vi "PathPlanner_ObstacleGrid_ReadNavFile.vi"(11 "FileName":string="default_navgrid.json") -> (0 "error out":errorcluster, 2 "NavGridObstacles":T1[](array[typedef]), 3 "PathPlanner_Grid":T2, 4 "Full Filename":string)   [LabVIEW 2019, in "PathPlanner24.lvlib"]
doc: "Load an obstacle grid from a JSON formatted file. \n\nInputs: \n - filename - string - The name of the obstacle grid file. See notes below on file naming.\n\nOutputs:\n - PathPlanner_ObstacleGrid - cluster - Obstacle grid read from JSON file.\n - Error out - cluster - Error cluster\n - Full Filename - string - fully qualified file name.\n\nNotes on file naming:\n - The file name must include the extention. \".json\" is not automatically appended to the name. \n - The file name can be a simple file or an absolute path. If a simple file name is used the default path on the RoboRIO is: \"home:\\lvuser\\natinst\\LabVIEW Data\". On a Windows PC the default path is the LabVIEW default directory. Normally this is: “%HOMEDRIVE%%HOMEPATH%\\Documents\\LabView Data\".\n - Filenames on the RoboRIO, which runs Linux, are case sensitive.\ni"
uses:
  PathPlanner24.lvlib
  TypeDef/PathPlannerObstacleGrid.ctl
  TypeDef/PathPlannerFinderGridPosition.ctl
panel:
  in  "error in (no error)":errorcluster
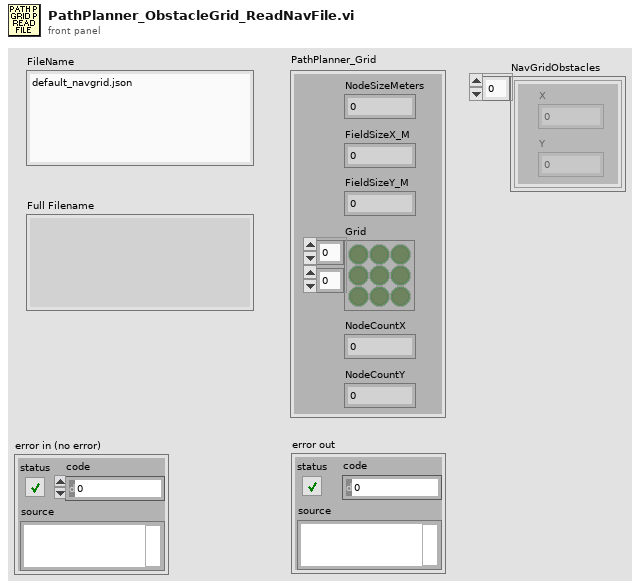
[diagram p1: front panel]
types:
  T1 = typedef "PathPlanner24.lvlib/PathPlannerFinderGridPosition.ctl" = cluster{"X":i32, "Y":i32}
  T2 = typedef "PathPlanner24.lvlib/PathPlannerObstacleGrid.ctl" = cluster{"NodeSizeMeters":dbl, "Grid":bool[][], "NodeCountX":i32, "NodeCountY":i32, "FieldSizeX_M":dbl, "FieldSizeY_M":dbl}
  T3 = enum16{"open", "replace", "create", "open or create", "replace or create", "replace or create with confirmation"}
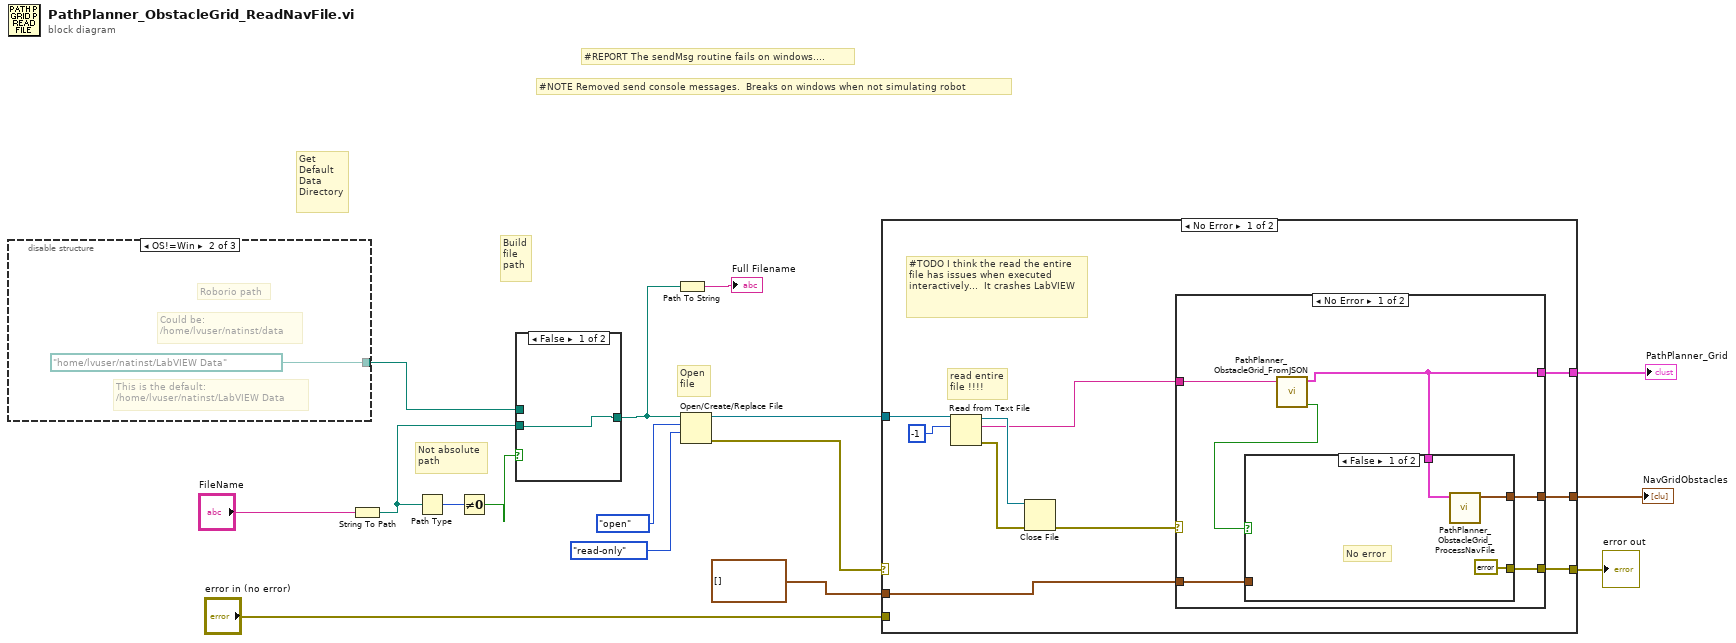
[diagram p0: block diagram]
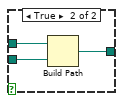
[diagram p2: hidden frame]
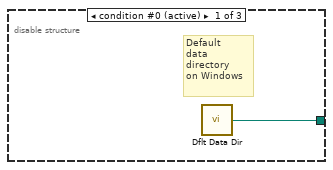
[diagram p3: hidden frame]
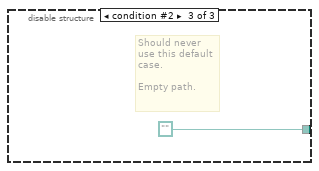
[diagram p4: hidden frame]
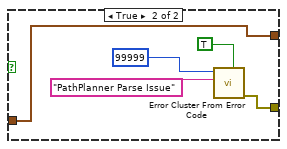
[diagram p5: hidden frame]
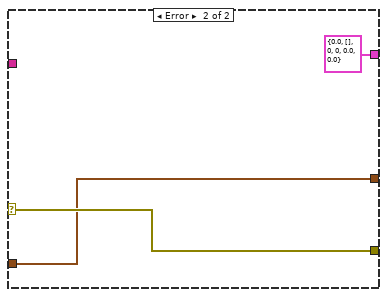
[diagram p6: hidden frame]
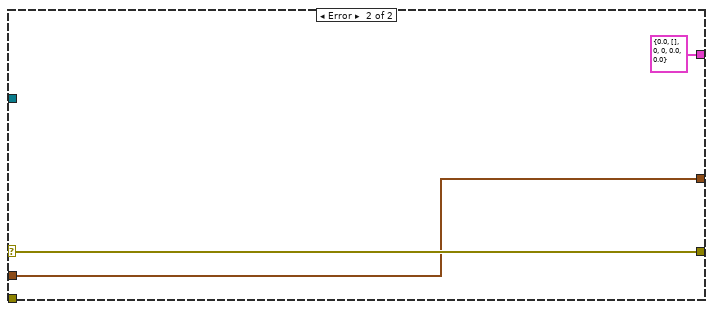
[diagram p7: hidden frame]
diagram:
  # "Not absolute\npath"
  # "#NOTE Removed send console messages.  Breaks on windows when not simulating robot"
  # "#REPORT The sendMsg routine fails on windows...."
  # "Get\nDefault\nData\nDirectory"
  # "Open\nfile"
  # "Build\nfile\npath"
  n1 = disable-structure shown="OS!=Win" {
    disable-tunnel: [w17 path "/home/lvuser/natinst/LabVIEW Data" path ""] -> w13
    frame condition #0 (active) {
      # "Default\ndata\ndirectory\non Windows"
      n2 = call <vilib>:"Dflt Data Dir.vi"() -> ("App:Default Data Directory"=w17:path)
    }
    frame condition #1 {
      # "This is the default:\n/home/lvuser/natinst/LabVIEW Data"
      # "Could be:\n/home/lvuser/natinst/data"
      # "Roborio path"
    }
    frame condition #2 {
      # "Should never\nuse this default\ncase.\n\nEmpty path."
    }
  }
  n3 = String To Path(string="FileName") -> (path=w12:path)
  n4 = Path Type(1:w12) -> (0:w11:i16)
  n5 = Not Equal To 0?(x=w11) -> (x != 0?=w10:bool)
  n6 = case shown="False" w10 {
    tunnel: [w20 w23] -> w7
    tunnel: w13 -> [_ w22]
    tunnel: w12 -> [w20 w21]
    frame False {
    }
    frame True {
      n7 = Build Path(base path=w22, name or relative path=w21) -> (appended path=w23:path)
    }
  }
  n8 = Path To String(path=w7) -> (string=→"Full Filename":string)
  n9 = Open/Create/Replace File(file path (use dialog)=w7, operation (0:open)=T3."open", access (0:read/write)=enum16{"read/write", "read-only", "write-only"}."read-only") -> (refnum out=w8:refnum<file>, error out=w14:errorcluster)  [unwired: 3 in, 1 out]
  n10 = case shown="No Error" w14 {
    selector: w14 -> [_ w53]
    tunnel: w8 -> [w32 _]
    tunnel: [w27 w53] -> w4
    tunnel: "error in (no error)" -> [_ _]
    tunnel: [w26 T2 {"NodeSizeMeters"=0.0, "Grid"=[], "NodeCountX"=0, "NodeCountY"=0, "FieldSizeX_M"=0.0, "FieldSizeY_M"=0.0} ("PathPlanner_Grid")] -> w3
    tunnel: [w25 w51] -> w2
    tunnel: T1[] [] ("NavGridObstacles") -> [w24 w51]
    frame No Error {
      # "#TODO I think the read the entire\nfile has issues when executed\ninteractively...  It crashes LabVIEW"
      # "read entire\nfile !!!!"
      n11 = Read from Text File(file (use dialog)=w32, count=-1) -> (refnum out=w31:refnum<file>, text=w30:string, error out=w29:errorcluster)  [unwired: 2 in, 1 out]
      n12 = Close File(refnum=w31, error in=w29) -> (error out=w28:errorcluster)  [unwired: 1 out]
      n13 = case shown="No Error" w28 {
        selector: w28 -> [_ w50]
        tunnel: w30 -> [w39 _]
        tunnel: [w37 w50] -> w27
        tunnel: [w36 T2 {"NodeSizeMeters"=0.0, "Grid"=[], "NodeCountX"=0, "NodeCountY"=0, "FieldSizeX_M"=0.0, "FieldSizeY_M"=0.0} ("PathPlanner_Grid")] -> w26
        tunnel: [w35 w48] -> w25
        tunnel: w24 -> [w34 w48]
        frame No Error {
          n14 = call "PathPlanner_ObstacleGrid_FromJSON.vi"("JSON String"=w39) -> ("Error"=w38:bool, "PathPlanner_Grid"=w36:T2)  [unwired: 9 in]
          n15 = case shown="False" w38 {
            tunnel: [errorcluster {"status"=FALSE, "code"=0, "source"=""} ("error out") w44] -> w37
            tunnel: w36 -> [w41 _]
            tunnel: [w40 w43] -> w35
            tunnel: w34 -> [_ w43]
            frame False {
              # "No error"
              n16 = call "PathPlanner_ObstacleGrid_ProcessNavFile.vi"("PathPlanner_Grid"=w41) -> ("NavGridObstacles"=w40:T1[])  [unwired: 10 in]
            }
            frame True {
              n17 = call <vilib>:"Error Cluster From Error Code.vi"("is warning? (False)"=TRUE, "error message (\"\")"="PathPlanner Parse Issue" ("error message (\"\")"), "error code (0)"=99999) -> ("error out"=w44:errorcluster)  [unwired: 6 in]
            }
          }
        }
        frame Error {
        }
      }
    }
    frame Error {
    }
  }
  "error out" <- w4
  "PathPlanner_Grid" <- w3
  "NavGridObstacles" <- w2
